vi "Starting Position and Angle.vi"() -> (0 "Angle":dbl, 2 "Location":cluster{"X":dbl, "Y":dbl})   [LabVIEW 2020]
uses:
  <vilib>/Rock Robotics/Network Tables/NT Read Number.vi
panel:
  in  "NT Override":bool
  in  "Position":dbl
  in  "Array":T1(array[cluster])=[{"Location"={"X"=0.0, "Y"=0.0}, "Angle"=0.0}, {"Location"={"X"=289.5, "Y"=127.4}, "Angle"=65.0}]
  # "LOCATIONS ARE 1 INDEXED!!!!! LOCATION 0 IS DEFAULT AND ALL 0's"
  # "Please leave NT Override as false when not using"
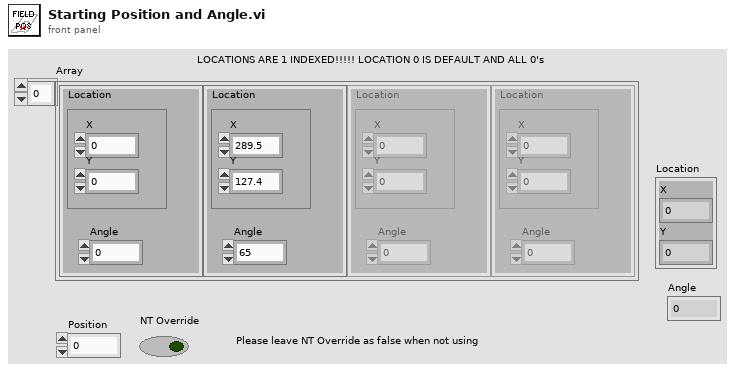
[diagram p1: front panel]
types:
  T1 = cluster{"Location":cluster{"X":dbl, "Y":dbl}, "Angle":dbl}[]
  T2 = cluster{"Location":cluster{"X":dbl, "Y":dbl}, "Angle":dbl}
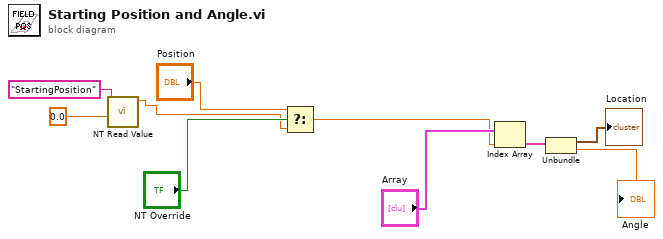
[diagram p0: block diagram]
diagram:
  n1 = call-poly <vilib>:"NT Read Value.vi"("Default Value"=0.0, "Name"="StartingPosition") -> ("Numeric"=w2:dbl)  [unwired: 8 in, 1 out]
  n2 = Select(t="Position", s="NT Override", f=w2) -> (s? t:f=w1:dbl)
  n3 = Index Array(array="Array", index=w1) -> (element=w7:T2)
  n4 = Unbundle(w7) -> ("Location"=→"Location":cluster{"X":dbl, "Y":dbl}, "Angle"=→"Angle":dbl)
